vi "Write Name.vi"(10 "Name":string, 11 "RelayInterface in":refnum<class "RelayInterface.lvclass">) -> (3 "RelayInterface out":refnum<class "RelayInterface.lvclass">)   [LabVIEW 2015, in "RelayInterface.lvclass"]
doc: "Write the name of this relay"
uses:
  RelayInterface.lvclass
  RelayInterface.lvclass/RelayInterface.ctl
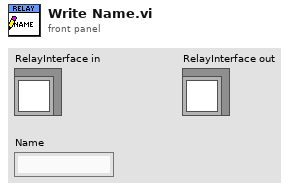
[diagram p1: front panel]
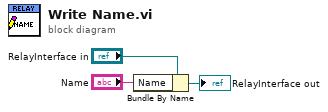
[diagram p0: block diagram]
diagram:
  n1 = Bundle By Name(cluster="RelayInterface in", "Name"="Name") -> (→"RelayInterface out":refnum<class "RelayInterface.lvclass">)
